vi "SwerveGlobals.vi"() -> ()   [LabVIEW 2018]
panel:
  in  "DriveMode":enum16{"Swerve", "Ackerman", ""}(ring)
  in  "ElevatorLvl":i16
  in  "?":bool
  in  "ZeroGyro":bool
  in  "HatchCatch":dbl
  in  "ClimbMode":bool
  in  "DropCargo":bool
  in  "Extend":bool
  in  "GyroOffset":dbl
  in  "Gyro":dbl
  in  "ZAxis":dbl
  in  "YAxis":dbl
  in  "XAxis":dbl
  # "Code:"
  # "Pilot:"
  # "Copilot:"
  # "Climb mode copilot:"
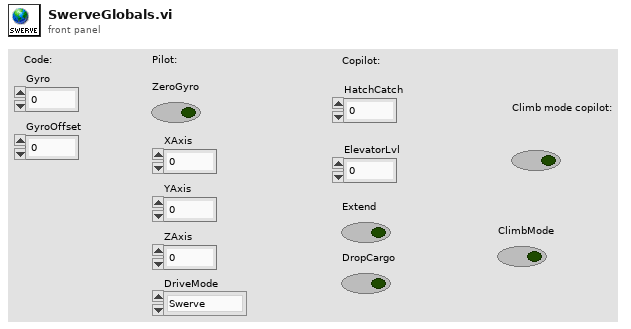
[diagram p1: front panel]
diagram:
